vi "centroid offset.vi"(9 "X_base":sgl, 10 "Y_base":sgl, 11 "Centroid XY输入":cluster{"X Centroid":sgl, "Y Centroid":sgl}) -> (3 "Centroid XY输出":cluster{"X Centroid":sgl, "Y Centroid":sgl})   [LabVIEW 2017]
doc: "本VI只是调试的时候使用的，用于将ROI提取后的图心坐标再进行补偿，得到实际上的图心坐标。\n在调试完毕后图心坐标已经无需显示了。"
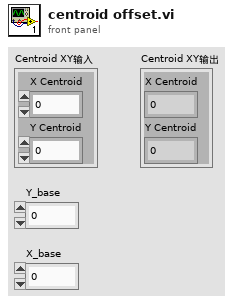
[diagram p1: front panel]
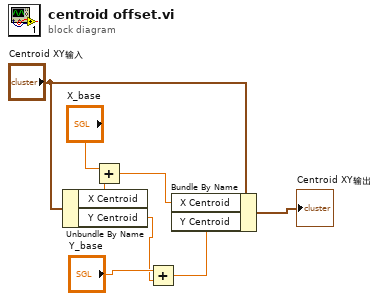
[diagram p0: block diagram]
diagram:
  n1 = Unbundle By Name("Centroid XY输入") -> ("X Centroid"=w1:sgl, "Y Centroid"=w4:sgl)
  n2 = Add(x="X_base", y=w1) -> (x+y=w3:sgl)
  n3 = Add(x="Y_base", y=w4) -> (x+y=w6:sgl)
  n4 = Bundle By Name(cluster="Centroid XY输入", "X Centroid"=w3, "Y Centroid"=w6) -> (→"Centroid XY输出":cluster{"X Centroid":sgl, "Y Centroid":sgl})
